vi "FindAddresses.vi"(0 "Toolbox in":refnum<class "Toolbox.lvclass">, 3 "error in (no error)":errorcluster) -> (7 "Toolbox out":refnum<class "Toolbox.lvclass">, 8 "Devices_Addressed":i32, 10 "error out":errorcluster)   [LabVIEW 2014, in "Driver_interaction.lvlib" / "Toolbox.lvclass"]
uses:
  Toolbox.lvclass
  _Driver_interaction/_Driver_interaction.lvclass
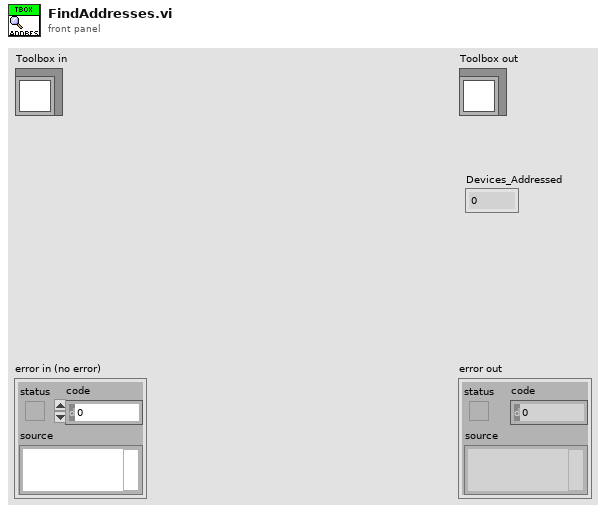
[diagram p1: front panel]
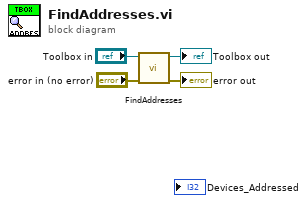
[diagram p0: block diagram]
diagram:
  n1 = call-parent "FindAddresses.vi"("_Driver_interaction in"="Toolbox in", "error in (no error)"="error in (no error)") -> ("_Driver_interaction out"=→"Toolbox out":refnum<class "Toolbox.lvclass">, "error out"=→"error out":errorcluster)  [unwired: 6 in, 1 out]
